vi "Get Line Name.vi"(8 "error in":errorcluster, 11 "Line in":T1={"Channel Array"=[], "Physical Channel"="", "Measurement Type"=enum."Digital Input", "Parameters"={"Digital Config"={"Invert Lines?"=FALSE}, "Voltage Config"={"Maximum Value (V)"=5.0, "Minimum Value (V)"=-5.0, "in terminal configuration (V)"=-1, "out terminal configuration (V)"=-1}, "Current Config"={"Maximum Value (A)"=0.02, "Minimum Value (A)"=0.0, "shunt resistor location"=-1, "input terminal configuration (C)"=-1, "external shunt resistor value"=249.0}, "RTD Config"={"Maximum Value (°C)"=100.0, "Minimum Value (°C)"=0.0, "resistance configuration"=2, "r0"=100.0, "current excitation value"=0.0025, "rtd type"=10137, "current excitation source"=10167}, "Thermocouple Config"={"Minimum Value (C)"=0.0, "Maximum Value (C)"=100.0, "thermocouple type"=10072, "cjc source"=10116, "cjc value"=25.0}, "Strain Config"={"Maximum Value"=0.001, "Minimum Value"=-0.001, "bridge information"={"strain configuration"=10183, "lead wire resistance"=0.0, "initial bridge voltage"=0.0, "voltage excitation source"=10200, "voltage excitation value"=2.5}, "strain gage information"={"gage factor"=2.0, "nominal gage resistance"=350.0, "poisson ratio"=0.3}}, "PWM Config"={"Idle State"=FALSE}}} {"Parameters"."Voltage Config"."out terminal configuration (V)" items=["Default"=-1, "RSE"=10083, "Differential"=10106, "Pseudodifferential"=12529]; "Parameters"."Voltage Config"."in terminal configuration (V)" items=["Default"=-1, "RSE"=10083, "NRSE"=10078, "Differential"=10106, "Pseudodifferential"=12529]; "Parameters"."Current Config"."shunt resistor location" items=["default"=-1, "Internal"=10200, "External"=10167]; "Parameters"."Current Config"."input terminal configuration (C)" items=["default"=-1, "RSE"=10083, "NRSE"=10078, "Differential"=10106, "Pseudodifferential"=12529]; "Parameters"."RTD Config"."resistance configuration" items=["2-Wire"=2, "3-Wire"=3, "4-Wire"=4]; "Parameters"."RTD Config"."rtd type" items=["Pt3750"=12481, "Pt3851"=10071, "Pt3911"=12482, "Pt3916"=10069, "Pt3920"=10053, "Pt3928"=12483, "Custom"=10137]; "Parameters"."RTD Config"."current excitation source" items=["Internal"=10200, "External"=10167, "None"=10230]; "Parameters"."Thermocouple Config"."thermocouple type" items=["J"=10072, "K"=10073, "N"=10077, "R"=10082, "S"=10085, "T"=10086, "B"=10047, "E"=10055]; "Parameters"."Thermocouple Config"."cjc source" items=["Built-In"=10200, "Constant Value"=10116, "Channel"=10113]; "Parameters"."Strain Config"."bridge information"."strain configuration" items=["Full Bridge I"=10183, "Full Bridge II"=10184, "Full Bridge III"=10185, "Half Bridge I"=10188, "Half Bridge II"=10189, "Quarter Bridge I"=10271, "Quarter Bridge II"=10272]; "Parameters"."Strain Config"."bridge information"."voltage excitation source" items=["Internal"=10200, "External"=10167, "None"=10230]}) -> (0 "error out":errorcluster, 2 "Name":string, 3 "Line out":T1={"Channel Array"=[], "Physical Channel"="", "Measurement Type"=enum."Digital Input", "Parameters"={"Digital Config"={"Invert Lines?"=FALSE}, "Voltage Config"={"Maximum Value (V)"=5.0, "Minimum Value (V)"=-5.0, "in terminal configuration (V)"=-1, "out terminal configuration (V)"=-1}, "Current Config"={"Maximum Value (A)"=0.02, "Minimum Value (A)"=0.0, "shunt resistor location"=-1, "input terminal configuration (C)"=-1, "external shunt resistor value"=249.0}, "RTD Config"={"Maximum Value (°C)"=100.0, "Minimum Value (°C)"=0.0, "resistance configuration"=2, "r0"=100.0, "current excitation value"=0.0025, "rtd type"=10137, "current excitation source"=10167}, "Thermocouple Config"={"Minimum Value (C)"=0.0, "Maximum Value (C)"=100.0, "thermocouple type"=10072, "cjc source"=10116, "cjc value"=25.0}, "Strain Config"={"Maximum Value"=0.001, "Minimum Value"=-0.001, "bridge information"={"strain configuration"=10183, "lead wire resistance"=0.0, "initial bridge voltage"=0.0, "voltage excitation source"=10200, "voltage excitation value"=2.5}, "strain gage information"={"gage factor"=2.0, "nominal gage resistance"=350.0, "poisson ratio"=0.3}}, "PWM Config"={"Idle State"=FALSE}}} {"Parameters"."Voltage Config"."out terminal configuration (V)" items=["Default"=-1, "RSE"=10083, "Differential"=10106, "Pseudodifferential"=12529]; "Parameters"."Voltage Config"."in terminal configuration (V)" items=["Default"=-1, "RSE"=10083, "NRSE"=10078, "Differential"=10106, "Pseudodifferential"=12529]; "Parameters"."Current Config"."shunt resistor location" items=["default"=-1, "Internal"=10200, "External"=10167]; "Parameters"."Current Config"."input terminal configuration (C)" items=["default"=-1, "RSE"=10083, "NRSE"=10078, "Differential"=10106, "Pseudodifferential"=12529]; "Parameters"."RTD Config"."resistance configuration" items=["2-Wire"=2, "3-Wire"=3, "4-Wire"=4]; "Parameters"."RTD Config"."rtd type" items=["Pt3750"=12481, "Pt3851"=10071, "Pt3911"=12482, "Pt3916"=10069, "Pt3920"=10053, "Pt3928"=12483, "Custom"=10137]; "Parameters"."RTD Config"."current excitation source" items=["Internal"=10200, "External"=10167, "None"=10230]; "Parameters"."Thermocouple Config"."thermocouple type" items=["J"=10072, "K"=10073, "N"=10077, "R"=10082, "S"=10085, "T"=10086, "B"=10047, "E"=10055]; "Parameters"."Thermocouple Config"."cjc source" items=["Built-In"=10200, "Constant Value"=10116, "Channel"=10113]; "Parameters"."Strain Config"."bridge information"."strain configuration" items=["Full Bridge I"=10183, "Full Bridge II"=10184, "Full Bridge III"=10185, "Half Bridge I"=10188, "Half Bridge II"=10189, "Quarter Bridge I"=10271, "Quarter Bridge II"=10272]; "Parameters"."Strain Config"."bridge information"."voltage excitation source" items=["Internal"=10200, "External"=10167, "None"=10230]})   [LabVIEW 2015, in "DAQmx Module Configuration.lvclass"]
doc: "This VI retrieves the line name or ID, that identifies this element in the cluster, from the line."
uses:
  Daqmx Module configuration.lvclass
  Line.ctl
  <vilib>/NI/Tag Bus Module Framework/channel/TBM channel.lvclass
  Measurement Type.ctl
  Parameters.ctl
  <vilib>/NI/Tag Bus/tag/tag descriptor.lvclass/tag descriptor.ctl
  <vilib>/NI/Tag Bus/tag/tag descriptor.lvclass
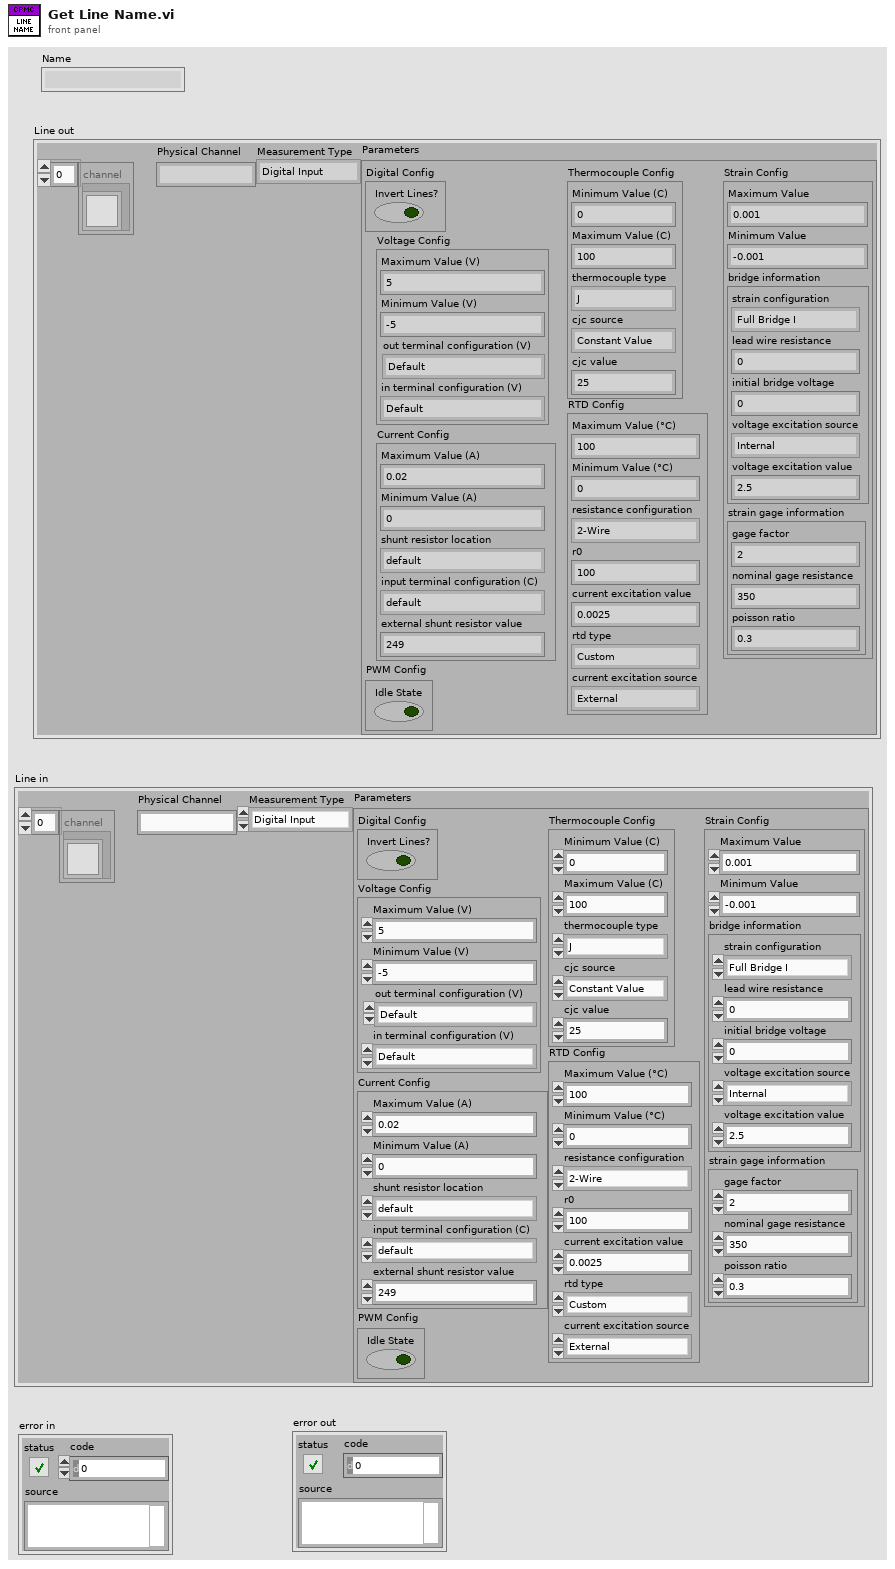
[diagram p1: front panel]
types:
  T1 = typedef "DAQmx Module Configuration.lvclass/Line.ctl" = cluster{"Channel Array":refnum<class "TBM channel.lvclass">[], "Physical Channel":string, "Measurement Type":T2, "Parameters":T3}
  T2 = typedef "DAQmx Module Configuration.lvclass/Measurement Type.ctl" = enum16{"Digital Input", "Digital Output", "Voltage Input", "Voltage Output", "Current Input", "Current Output", "RTD", "Thermocouple", "Strain", "PWM"}
  T3 = typedef "DAQmx Module Configuration.lvclass/Parameters.ctl" = cluster{"Digital Config":cluster{"Invert Lines?":bool}, "Voltage Config":cluster{"Maximum Value (V)":dbl, "Minimum Value (V)":dbl, "in terminal configuration (V)":i32, "out terminal configuration (V)":i32}, "Current Config":cluster{"Maximum Value (A)":dbl, "Minimum Value (A)":dbl, "shunt resistor location":i32, "input terminal configuration (C)":i32, "external shunt resistor value":dbl}, "RTD Config":cluster{"Maximum Value (°C)":dbl, "Minimum Value (°C)":dbl, "resistance configuration":i32, "r0":dbl, "current excitation value":dbl, "rtd type":i32, "current excitation source":i32}, "Thermocouple Config":cluster{"Minimum Value (C)":dbl, "Maximum Value (C)":dbl, "thermocouple type":i32, "cjc source":i32, "cjc value":dbl}, "Strain Config":cluster{"Maximum Value":dbl, "Minimum Value":dbl, "bridge information":cluster{"strain configuration":i32, "lead wire resistance":dbl, "initial bridge voltage":dbl, "voltage excitation source":i32, "voltage excitation value":dbl}, "strain gage information":cluster{"gage factor":dbl, "nominal gage resistance":dbl, "poisson ratio":dbl}}, "PWM Config":cluster{"Idle State":bool}}
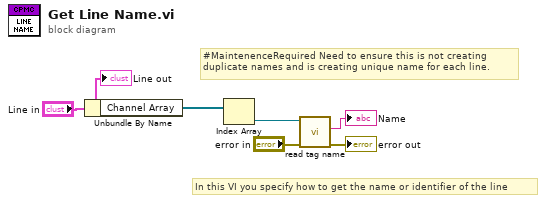
[diagram p0: block diagram]
diagram:
  # "#MaintenenceRequired Need to ensure this is not creating\nduplicate names and is creating unique name for each line."
  # "In this VI you specify how to get the name or identifier of the line"
  n1 = Unbundle By Name("Line in") -> ("Channel Array"=w1:refnum<class "TBM channel.lvclass">[])
  n2 = Index Array(array=w1) -> (element=w2:refnum<class "TBM channel.lvclass">)  [unwired: 1 in]
  n3 = call <vilib>:"read tag name.vi"("error in"="error in", "system tag in"=w2) -> ("error out"=→"error out":errorcluster, "name"=→"Name":string)  [unwired: 7 in, 1 out]
  "Line out" <- "Line in"
